vi "Deserialize JSON to LabVIEW Object Base Class.vi"() -> ()   [LabVIEW 2020]
doc: "This VI demonstrates a function of the GCraftsman JSON Serialization Toolkit.\n\nIt uses the 'Unflatten from JSON String' function to deserialize a JSON string into a LabVIEW object. Since type information is included in the JSON string, the 'Unflatten' function doesn't require a specific instance type to be wired to it. Here it is simply using 'LabVIEW Object' - the common ancestor datatype for all LabVIEW Classes.\n\nThis does not require the classes to have accessor methods.\n\nGCraftsman JSON Object Serialization Toolkit\nwww.GCraftsman.com\nCopyright (c) 2017, GCraftsman"
uses:
  Class3/Class3.lvclass
  Class2/Class2.lvclass
  library/JKI JSON Object Serialization.lvlib
panel:
  out "myBool":bool
  out "anotherNumber":dbl format="%#_13g"
  out "someNumber":dbl format="%#_13g"
  out "myNum 2":dbl format="%#_13g"
  out "myNum":dbl format="%#_13g"
  out "unflattenedObj":refnum<class "Class2.lvclass">
  in  "JSON String":string="{\r\n    \"@type\":\"Class2.lvclass\",\r\n    \"someNumber\":456,\r\n    \"myClass3Array\":[\r\n        {\r\n            \"@type\":\"Class3.lvclass\",\r\n            \"myNum\":444\r\n        },\r\n        {\r\n            \"@type\":\"Class3.lvclass\",\r\n            \"myNum\":555\r\n        }\r\n    ],\r\n    \"myBool\":true,\r\n    \"anotherNumber\":123\r\n}"
  # "This VI demonstrates a function of the GCraftsman JSON Serialization Toolkit.\n\nLook at the block diagram to see that the 'Unflatten from JSON String' function can deserialize a JSON string into a LabVIEW object.   Since '@type' information is included in the JSON string, the 'Unflatten' function doesn't require a specific instance type to be wired to it.  Here it is simply using 'LabVIEW Object' - the common ancestor datatype for all LabVIEW Classes.\n\nRun this VI ."
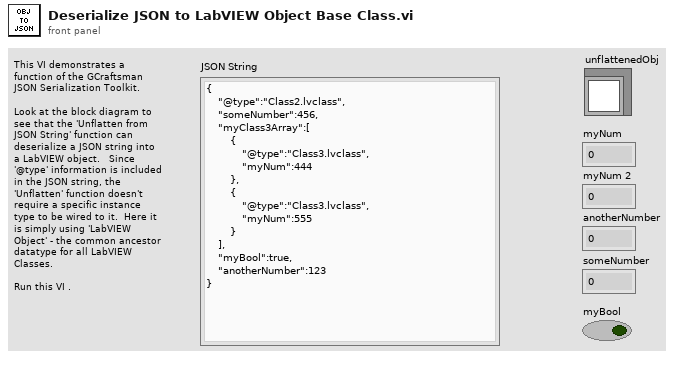
[diagram p1: front panel]
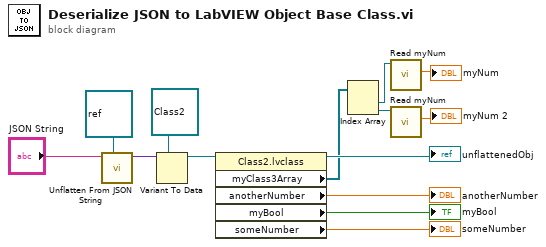
[diagram p0: block diagram]
diagram:
  n1 = call "Unflatten From JSON String.vi"("Type and Defaults"=refnum<class> refnum ("LabVIEW Object"), "JSON String"="JSON String") -> ("Variant"=w4:variant)  [unwired: 8 in, 1 out]
  n2 = Variant To Data(type=refnum<class "Class2.lvclass"> refnum ("reference"), Variant=w4) -> (data=w3:refnum<class "Class2.lvclass">)  [unwired: 1 in, 1 out]
  n3 = property class="Class2.lvclass"(reference=w3) -> (reference out=→"unflattenedObj":refnum<class "Class2.lvclass">, "myClass3Array"=w9:refnum<class "Class3.lvclass">[], "anotherNumber"=→"anotherNumber":dbl, "myBool"=→"myBool":bool, "someNumber"=→"someNumber":dbl)  [unwired: 1 in, 1 out]
  n4 = Index Array(array=w9) -> (element #1=w14:refnum<class "Class3.lvclass">, element #2=w13:refnum<class "Class3.lvclass">)  [unwired: 2 in]
  n5 = call "Read myNum.vi"("Class3 in"=w14) -> ("myNum"=→"myNum":dbl)  [unwired: 8 in, 2 out]
  n6 = call "Read myNum.vi"("Class3 in"=w13) -> ("myNum"=→"myNum 2":dbl)  [unwired: 8 in, 2 out]
